vi "GitPathList.vi"(8 "error in (no error)":errorcluster, 11 "GitCheckFileList":path=path "C:/RageATE/Automated Tests/Tetra WAM/PRODUCTION/Test Benches/Common/Git_CheckList.txt") -> (0 "error out":errorcluster, 3 "pathlist_out":path[](array[path]))   [LabVIEW 2018]
uses:
  <vilib>/Utility/file.llb/Read Delimited Spreadsheet (string).vi
panel:
  # "Open the Git list of directories to check and send out as path(s)"
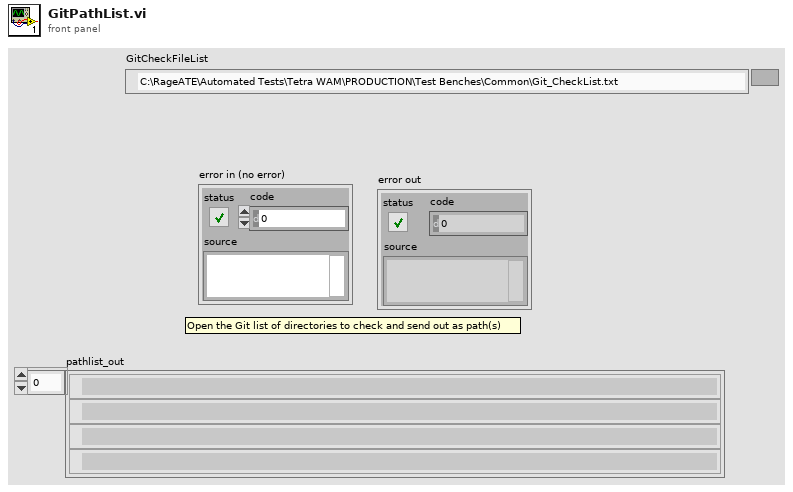
[diagram p1: front panel]
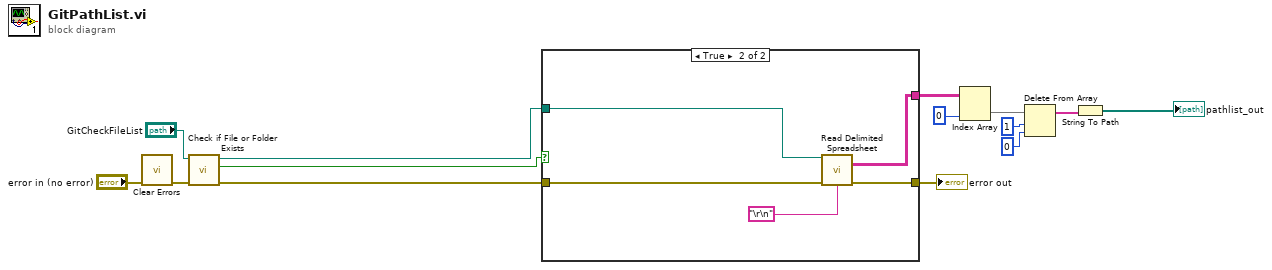
[diagram p0: block diagram]
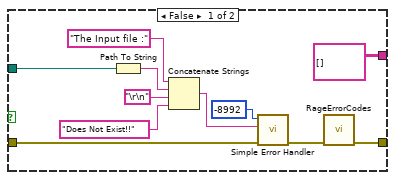
[diagram p2: hidden frame]
diagram:
  n1 = call <vilib>:"Clear Errors.vi"("error in (no error)"="error in (no error)") -> ("error out"=w5:errorcluster)  [unwired: 5 in, 1 out]
  n2 = call <vilib>:"Check if File or Folder Exists.vi"("error in (no error)"=w5, "path"="GitCheckFileList") -> ("error out"=w6:errorcluster, "file or folder exists?"=w8:bool, "dup path"=w7:path)  [unwired: 7 in]
  n3 = case shown="True" w8 {
    tunnel: [string[][] [] ("all rows") w30] -> w14
    tunnel: w6 -> [w16 w29]
    tunnel: [w19 w28] -> w10
    tunnel: w7 -> [w25 w27]
    frame False {
      n4 = Path To String(path=w25) -> (string=w23:string)
      n5 = Concatenate Strings("The Input file :", w23, "\r\n", "Does Not Exist!!" ("string")) -> (w15:string)
      n6 = call <vilib>:"Simple Error Handler.vi"("error code (no error:0)"=-8992, "error source (\" \")"=w15, "error in (no error)"=w16) -> ("error out"=w18:errorcluster)  [unwired: 2 in, 4 out]
      n7 = call "RageErrorCodes.vi"("error in"=w18) -> ("error out"=w19:errorcluster)  [unwired: 8 in, 2 out]
    }
    frame True {
      n8 = call-poly <vilib>:"Read Delimited Spreadsheet.vi"("file path (dialog if empty)"=w27, "error in (no error)"=w29, "delimiter (\\t)"="\r\n") -> ("all rows"=w30:string[][], "error out"=w28:errorcluster)  [unwired: 7 in, 4 out]
    }
  }
  "error out" <- w10
  n9 = Index Array(array=w14, index (col)=0 ("disabled index (col)")) -> (element=w13:string[])  [unwired: 1 in]
  n10 = Delete From Array(array=w13, length=1, index=0) -> (array with subset deleted=w1:string[])  [unwired: 1 out]
  n11 = String To Path(string=w1) -> (path=→"pathlist_out":path[])
